vi "New Button.vi"(11 "theme path":path=path "C:/Users/daniel.coons/Downloads/tsc-theme.xml") -> (0 "error out":errorcluster)   [LabVIEW 2021]
uses:
  Material Theme.lvclass/Material Theme.ctl
  Material Theme.lvclass
  Material-Scheme/Material-Scheme.lvclass
panel:
  in  "Path to Saved File":path=path "C:/Development/Reuse-libraries/_pics/button--save.ctl"
  in  "template":path=path "C:/Development/Reuse-libraries/TSC Material Theme/controls/nooutline--icon--rectangular--40x40.ctl"
  in  "Replace Image":path=path "C:/Users/daniel.coons/Downloads/save_FILL0_wght300_GRAD200_opsz40.png"
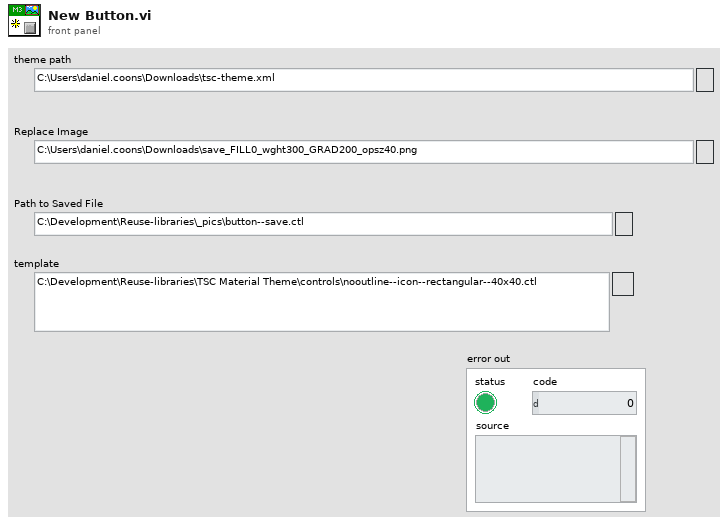
[diagram p1: front panel]
types:
  T1 = enum32{"invalid VI type", "Standard VI", "Control VI", "Global VI", "Polymorphic VI", "Configuration VI", "SubSystem", "Facade VI", "Method VI", "Statechart Diagram VI"}
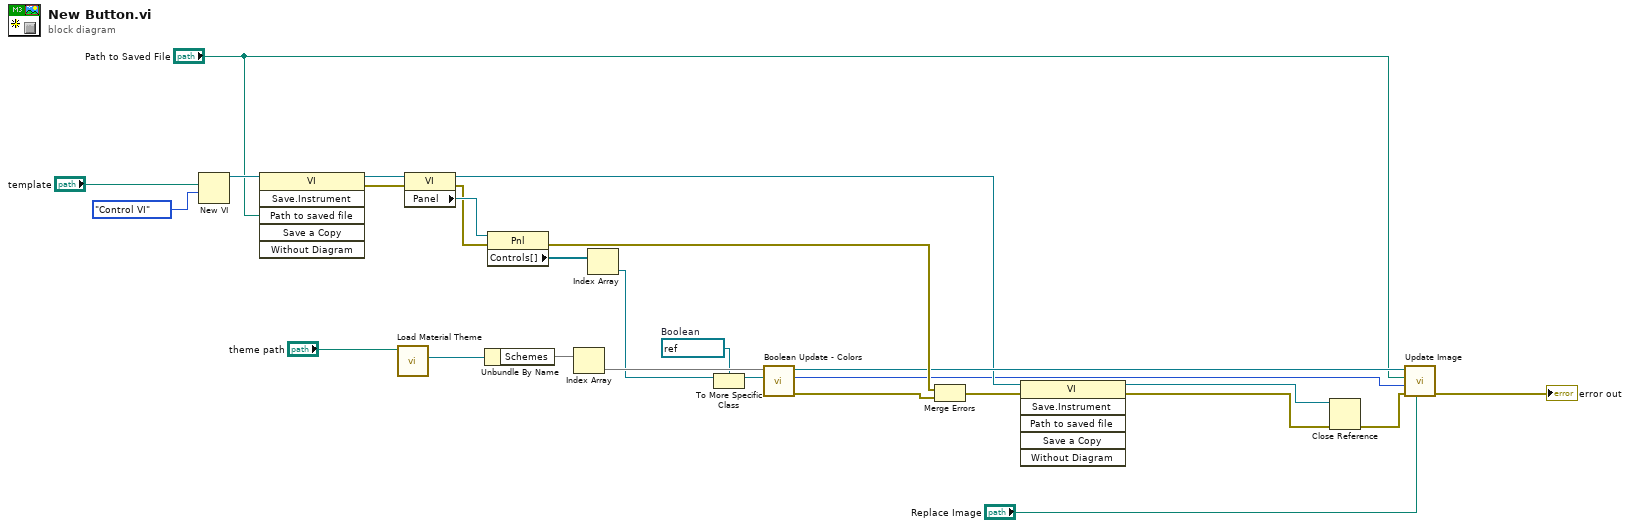
[diagram p0: block diagram]
diagram:
  w3 = refnum<vi> refnum  # Boolean
  n1 = New VI(9:T1."Control VI" ("vi type (standard vi)"), 10:"template") -> (3:w25:refnum<vi>)  [unwired: 5 in, 1 out]
  n2 = invoke class="VI" method="Save.Instrument"(reference=w25, "Path to saved file"="Path to Saved File") -> (reference out=w17:refnum<vi>, error out=w15:errorcluster)  [unwired: 4 in, 4 out]
  n3 = call "Load Material Theme.vi"("file path (use dialog)"="theme path") -> ("Theme"=w21:refnum<class "Material Theme.lvclass">)  [unwired: 9 in, 1 out]
  n4 = property class="VI"(reference=w17, error in=w15) -> (reference out=w8:refnum<vi>, error out=w14:errorcluster, "Panel"=w24:refnum<vi>)
  n5 = Unbundle By Name(w21) -> ("Schemes"=w20)
  n6 = property class="Pnl"(reference=w24, error in=w14) -> (error out=w12:errorcluster, "Controls[]"=w23:refnum<vi>[])  [unwired: 1 out]
  n7 = Index Array(array=w20) -> (element=w19)  [unwired: 1 in]
  n8 = Index Array(array=w23) -> (element=w18:refnum<vi>)  [unwired: 1 in]
  n9 = To More Specific Class(target class=w3, reference=w18) -> (specific class reference=w4:refnum<vi>)  [unwired: 1 in, 1 out]
  n10 = call "Boolean Update - Colors.vi"("Bool Refnum"=w4, "Material-Scheme in"=w19) -> ("error out"=w16:errorcluster, "font color"=w1:u32, "Material-Scheme"=w10:refnum<class "Material-Scheme.lvclass">)  [unwired: 6 in, 1 out]
  n11 = Merge Errors(w12, w16) -> (w13:errorcluster)
  n12 = invoke class="VI" method="Save.Instrument"(reference=w8, error in=w13) -> (reference out=w6:refnum<vi>, error out=w11:errorcluster)  [unwired: 4 in, 4 out]
  n13 = Close Reference(reference=w6, error in (no error)=w11) -> (error out=w7:errorcluster)
  n14 = call "Update Image.vi"("Replace Image"="Replace Image", "error in"=w7, "New Color"=w1, "New Control"="Path to Saved File", "Material-Scheme.lvclass"=w10) -> ("error out"=→"error out":errorcluster)  [unwired: 5 in, 1 out]
